vi "add channel.vi"(8 "error in (no error)":errorcluster, 10 "channel":refnum<class "TBM channel.lvclass">, 11 "E2E configuration in":refnum<class "E2E Tag Exchange configuration.lvclass">) -> (0 "error out":errorcluster, 3 "E2E configuration out":refnum<class "E2E Tag Exchange configuration.lvclass">)   [LabVIEW 2015, in "E2E Tag Exchange configuration.lvclass"]
uses:
  E2E Tag Exchange configuration.lvclass
  <vilib>/NI/Tag Bus Module Framework/channel/TBM channel.lvclass
  E2E Tag Exchange configuration.lvclass/E2E Tag Exchange configuration.ctl
  <vilib>/NI/Tag Bus/tag/tag descriptor.lvclass/tag descriptor.ctl
  <vilib>/NI/Tag Bus/tag/tag descriptor.lvclass
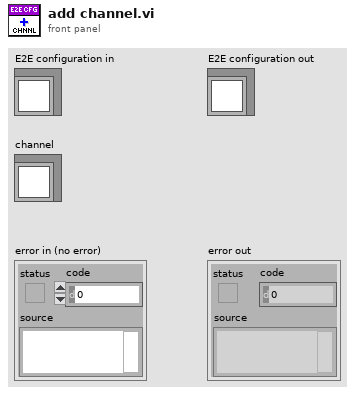
[diagram p1: front panel]
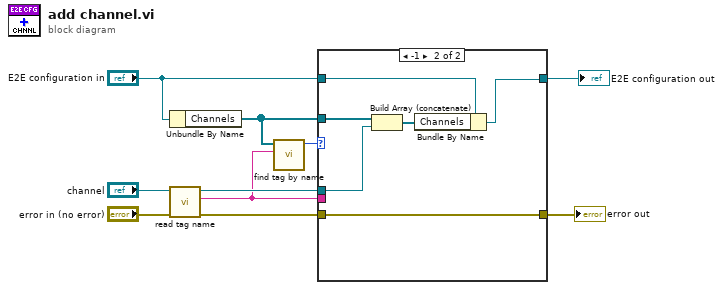
[diagram p0: block diagram]
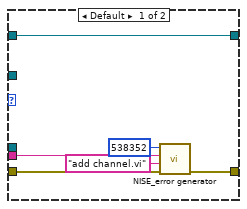
[diagram p2: hidden frame]
diagram:
  n1 = Unbundle By Name("E2E configuration in") -> ("Channels"=w6:refnum<class "TBM channel.lvclass">[])
  n2 = call <vilib>:"read tag name.vi"("error in"="error in (no error)", "system tag in"="channel") -> ("error out"=w4:errorcluster, "name"=w1:string, "system tag out"=w7:refnum<class "TBM channel.lvclass">)  [unwired: 7 in]
  n3 = call <vilib>:"find tag by name.vi"("name"=w1, "tags in"=w6) -> ("index"=w9:i32)  [unwired: 9 in]
  n4 = case shown="-1" w9 {
    tunnel: "E2E configuration in" -> [w16 w22]
    tunnel: w7 -> [_ w19]
    tunnel: w6 -> [_ w21]
    tunnel: w4 -> [w15 w18]
    tunnel: [w14 w18] -> w3
    tunnel: [w16 w17] -> w2
    tunnel: w1 -> [w12 _]
    frame Default {
      n5 = call <vilib>:"NISE_error generator.vi"("error in"=w15, "source"="add channel.vi", "append error message"=w12, "error code (0)"=538352) -> ("error out"=w14:errorcluster)  [unwired: 5 in]
    }
    frame -1 {
      n6 = Build Array (concatenate)(w21, w19) -> (w20:refnum<class "TBM channel.lvclass">[])
      n7 = Bundle By Name(cluster=w22, "Channels"=w20) -> (w17:refnum<class "E2E Tag Exchange configuration.lvclass">)
    }
  }
  "error out" <- w3
  "E2E configuration out" <- w2
